vi "Add_Log_File_Comment_client.vi"(1 "Comments to Add to the Log files":string) -> ()   [LabVIEW 2010]
doc: "This is an example of using features of the VI Server as a client. It shows how you might browse from one or more applications that may be exporting data from one or more data stations. \n\nThe example shows how to query a server for its list of exported VIs, how to get references to the VIs, and how call them with the Call By Reference function."
uses:
  Anemometry/Anemometry Sub Vis/Globals/Preference_global.vi
panel:
  in  "Server type":refnum<vi>
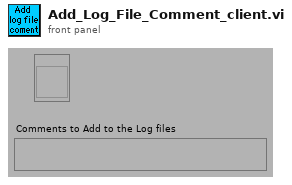
[diagram p1: front panel]
types:
  T1 = typedef "Server_Comms.ctl" = enum16{"Server Link Healthy", "Do Not Link To Server"}
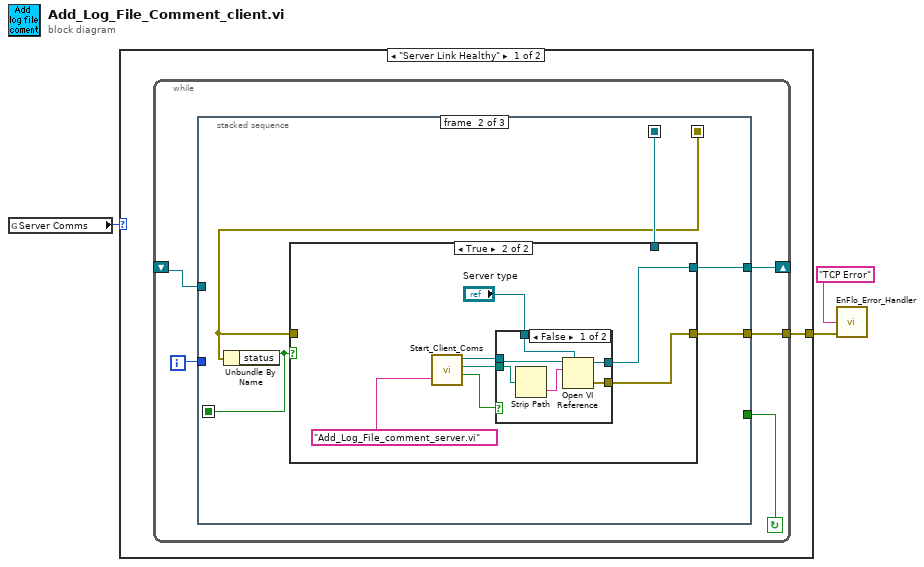
[diagram p0: block diagram]
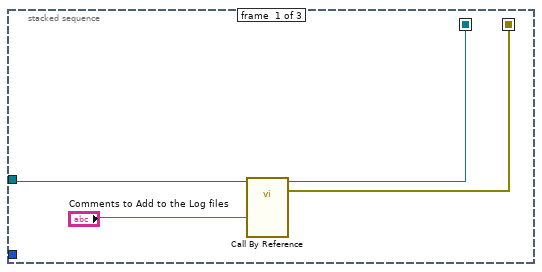
[diagram p2: hidden frame]
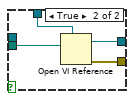
[diagram p4: hidden frame]
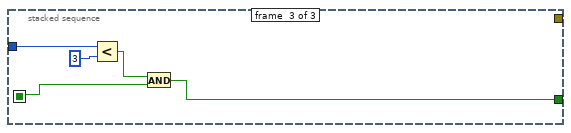
[diagram p5: hidden frame]
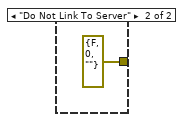
[diagram p6: hidden frame]
diagram:
  n1 = global read "Preference_global.vi" "Server Comms"() -> (w3:T1)
  n2 = case shown="\"Server Link Healthy\"" w3 {
    tunnel: [w4 errorcluster {"status"=FALSE, "code"=0, "source"=""} ("Error IO")] -> w2
    frame "Server Link Healthy" {
      n3 = while {
        tunnel: [w5] -> w4
        shift-left: _ -> [w9]
        shift-right: [w8] -> _
        i -> [w7]
        stop <- w6 continue-if-true
        n4 = stacked-sequence {
          seq-local: [w12 _ _] -> [_ w17 _]
          seq-local: [w11 _ _] -> [_ w14 _]
          seq-local: [_ w16 _] -> [_ _ w39]
          tunnel: w9 -> [w13 _ _]
          tunnel: [_ w18 _] -> w8
          tunnel: w7 -> [_ _ w40]
          tunnel: [_ _ w38] -> w6
          tunnel: [_ w15 _] -> w5
          frame #0 {
            n5 = call-by-ref "?"(reference=w13, "Comments to Add to the Log files"="Comments to Add to the Log files") -> (reference out=w12:refnum<vi>, error out=w11:errorcluster)  [unwired: 1 in]
          }
          frame #1 {
            n6 = Unbundle By Name(w14) -> ("status"=w16:bool)
            n7 = case shown="True" w16 {
              tunnel: [w20 w23] -> w18
              tunnel: w17 -> [w20 _]
              tunnel: [w19 w21] -> w15
              tunnel: w14 -> [w19 _]
              frame False {
              }
              frame True {
                n8 = call "Start_Client_Coms.vi"("VI name to run on server"="Add_Log_File_comment_server.vi") -> ("LabVIEW application reference"=w25:refnum<vi>, "Checked VI name"=w26:path, "Local Call"=w24:bool)  [unwired: 1 in, 1 out]
                n9 = case shown="False" w24 {
                  tunnel: [w29 w37] -> w23
                  tunnel: "Server type" -> [w30 w36]
                  tunnel: w26 -> [w33 w34]
                  tunnel: w25 -> [w31 _]
                  tunnel: [w28 w35] -> w21
                  frame False {
                    n10 = Strip Path(path=w33) -> (name=w32:string)  [unwired: 1 out]
                    n11 = Open VI Reference(type specifier VI Refnum (for type only)=w30, application reference (local)=w31, vi path=w32) -> (vi reference=w29:refnum<vi>, error out=w28:errorcluster)  [unwired: 1 in, 2 out]
                  }
                  frame True {
                    n12 = Open VI Reference(type specifier VI Refnum (for type only)=w36, vi path=w34) -> (vi reference=w37:refnum<vi>, error out=w35:errorcluster)  [unwired: 1 in, 3 out]
                  }
                }
              }
            }
          }
          frame #2 {
            n13 = Less?(x=w40, y=3) -> (x < y?=w42:bool)
            n14 = And(x=w42, y=w39) -> (x .and. y?=w38:bool)
          }
        }
      }
    }
    frame "Do Not Link To Server" {
    }
  }
  n15 = call "EnFlo_Error_Handler.vi"("error in (no error)"=w2, "Error Type"="TCP Error") -> ()  [unwired: 1 in, 3 out]
